vi "CreateClasses.vi"(8 "error in":errorcluster, 11 "PythonConverter_BD in":refnum<class "PyConvBD.lvclass">) -> (0 "error out":errorcluster, 3 "PythonConverter_BD out":refnum<class "PyConvBD.lvclass">)   [LabVIEW 2014, in "PyConvBD.lvclass"]
uses:
  PyConvBD.lvclass
  PyConvBD.lvclass/PyConvBD.ctl
  VI Interpreter/Classes/VI Interpreter/VI Interpreter.lvclass
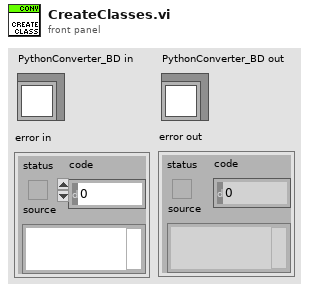
[diagram p1: front panel]
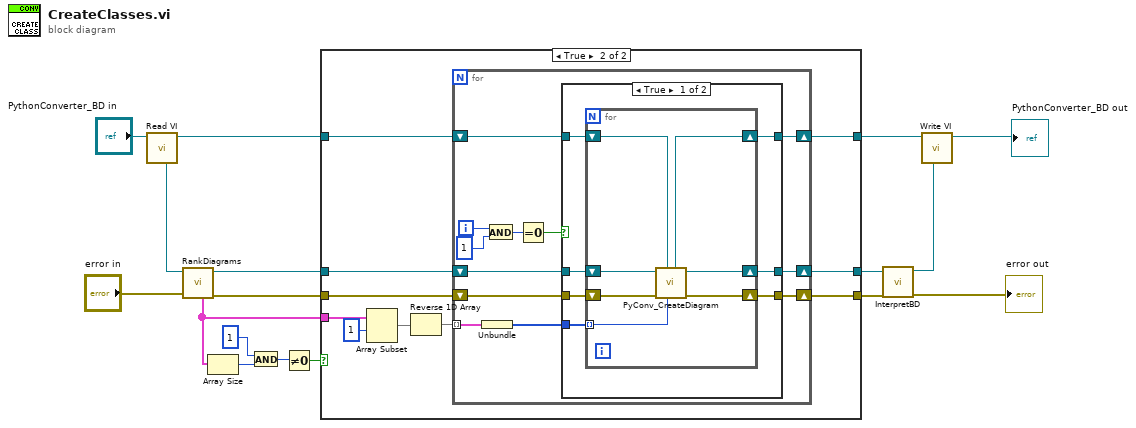
[diagram p0: block diagram]
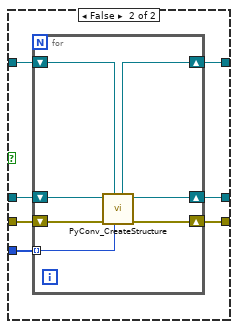
[diagram p3: hidden frame]
diagram:
  n1 = call "Read VI.vi"("PythonConverter_BD in"="PythonConverter_BD in") -> ("PythonConverter_BD out"=w13:refnum<class "PyConvBD.lvclass">, "VI Interpreter"=w12:refnum<class "VI Interpreter.lvclass">)  [unwired: 7 in]
  n2 = call "RankDiagrams.vi"("error in"="error in", "VI Interpreter in"=w12) -> ("error out"=w11:errorcluster, "VI Interpreter out"=w9:refnum<class "VI Interpreter.lvclass">, "Rank"=w10:cluster{"nodes":i32[]}[])  [unwired: 5 in]
  n3 = Array Size(array=w10) -> (size(s)=w5:i32)
  n4 = And(x=1, y=w5) -> (x .and. y?=w7:i32)
  n5 = Not Equal To 0?(x=w7) -> (x != 0?=w8:bool)
  n6 = case shown="True" w8 {
    tunnel: w9 -> [w19 w27]
    tunnel: w10 -> [_ w30]
    tunnel: w11 -> [w18 w26]
    tunnel: w13 -> [w20 w24]
    tunnel: [w20 w23] -> w14
    tunnel: [w19 w22] -> w16
    tunnel: [w18 w21] -> w15
    frame False {
    }
    frame True {
      n7 = Array Subset(array=w30, index=1) -> (w28:cluster{"nodes":i32[]}[])  [unwired: 1 in]
      n8 = Reverse 1D Array(array=w28) -> (reversed array=w25:cluster{"nodes":i32[]}[])
      n9 = for {
        shift-right: [w36] -> w22
        shift-left: w27 -> [w39]
        shift-right: [w35] -> w21
        shift-left: w26 -> [w37]
        tunnel: w25 -> [w32] mode=indexing
        shift-right: [w33] -> w23
        shift-left: w24 -> [w34]
        i -> [w42]
        n10 = Unbundle(w32) -> ("nodes"=w31:i32[])
        n11 = And(x=w42, y=1) -> (x .and. y?=w40:i32)
        n12 = Equal To 0?(x=w40) -> (x = 0?=w38:bool)
        n13 = case shown="True" w38 {
          tunnel: w39 -> [w49 w63]
          tunnel: w37 -> [w48 w62]
          tunnel: [w47 w61] -> w36
          tunnel: [w46 w60] -> w35
          tunnel: w34 -> [w45 w59]
          tunnel: [w44 w58] -> w33
          tunnel: w31 -> [w43 w57]
          frame True {
            n14 = for {
              tunnel: w43 -> [w50] mode=indexing
              shift-right: [w54] -> w47
              shift-left: w49 -> [w56]
              shift-right: [w53] -> w46
              shift-left: w48 -> [w55]
              shift-right: [w51] -> w44
              shift-left: w45 -> [w52]
              n15 = call "PyConv_CreateDiagram.vi"("UID"=w50, "PythonConverter_BD in"=w52, "error in"=w55, "VI Interpreter in"=w56) -> ("error out"=w53:errorcluster, "VI Interpreter out"=w54:refnum<class "VI Interpreter.lvclass">, "PythonConverter_BD out"=w51:refnum<class "PyConvBD.lvclass">)  [unwired: 5 in]
            }
          }
          frame False {
            n16 = for {
              tunnel: w57 -> [w65] mode=indexing
              shift-right: [w68] -> w61
              shift-left: w63 -> [w70]
              shift-right: [w67] -> w60
              shift-left: w62 -> [w69]
              shift-right: [w64] -> w58
              shift-left: w59 -> [w66]
              n17 = call "PyConv_CreateStructure.vi"("UID"=w65, "PythonConverter_BD in"=w66, "error in"=w69, "VI Interpreter in"=w70) -> ("error out"=w67:errorcluster, "VI Interpreter out"=w68:refnum<class "VI Interpreter.lvclass">, "PythonConverter_BD out"=w64:refnum<class "PyConvBD.lvclass">)  [unwired: 5 in]
            }
          }
        }
      }
    }
  }
  n18 = call "InterpretBD.vi"("error in"=w15, "VI Interpreter in"=w16) -> ("error out"=→"error out":errorcluster, "VI Interpreter out"=w17:refnum<class "VI Interpreter.lvclass">)  [unwired: 6 in]
  n19 = call "Write VI.vi"("VI Interpreter"=w17, "PythonConverter_BD in"=w14) -> ("PythonConverter_BD out"=→"PythonConverter_BD out":refnum<class "PyConvBD.lvclass">)  [unwired: 7 in]
